vi "VAT.vi"(2 "Разность":dbl, 3 "Temper":dbl, 4 "Атмосферное":dbl, 5 "Вип":dbl) -> (0 "n":dbl, 1 "раз":dbl)   [LabVIEW 2018]
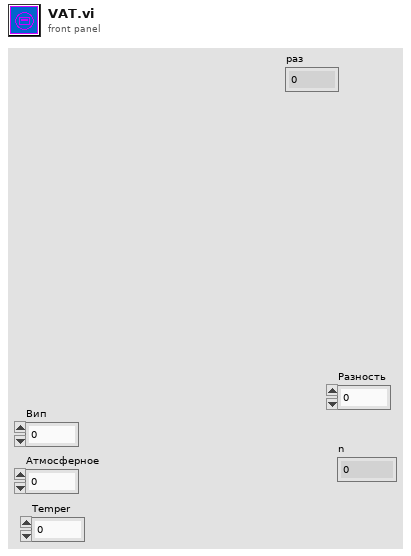
[diagram p1: front panel]
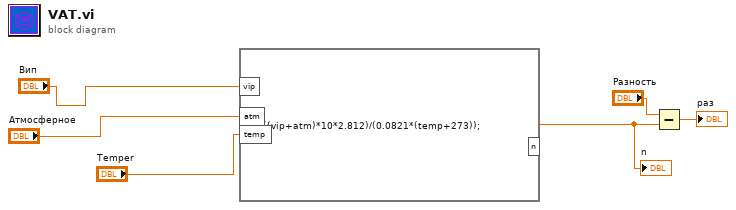
[diagram p0: block diagram]
diagram:
  n1 = formula code="n=((vip+atm)*10*2.812)/(0.0821*(temp+273));"("vip"="Вип", "atm"="Атмосферное", "temp"="Temper") -> ("n"=w2:dbl)
  "n" <- w2
  n2 = Subtract(x="Разность", y=w2) -> (x-y=→"раз":dbl)
